vi "writeU16FIFO.vi"(8 "error in (no error)":errorcluster, 9 "Timeout":i32, 10 "Data":u16[](array[numeric]), 11 "ModbusSubnetETxDataFIFO in":refnum<class "ModbusSubnetETxDataFIFO.lvclass">) -> (0 "error out":errorcluster, 2 "ElementsRemaining":u32, 3 "ModbusSubnetETxDataFIFO out":refnum<class "ModbusSubnetETxDataFIFO.lvclass">)   [LabVIEW 2016, in "ModbusSubnetETxDataFIFO.lvclass"]
uses:
  ModbusSubnetETxDataFIFO.lvclass
  FPGA/FPGA.lvclass
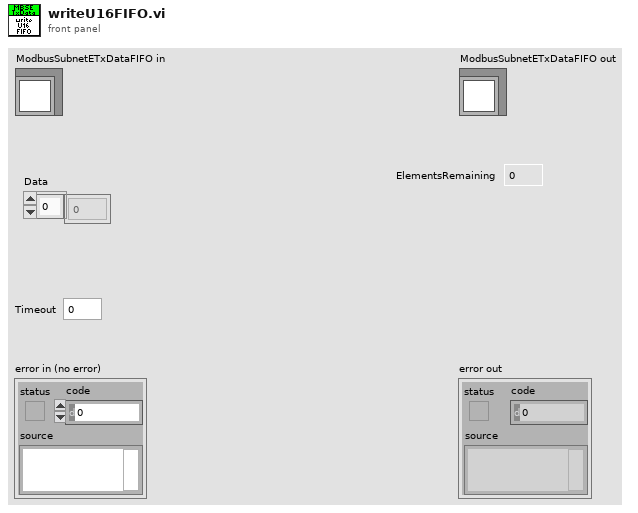
[diagram p1: front panel]
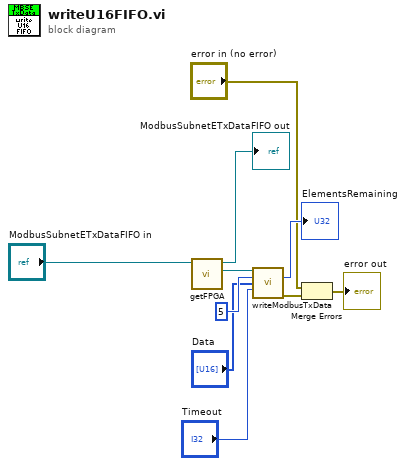
[diagram p0: block diagram]
diagram:
  n1 = call "getFPGA.vi"("ModbusSubnetETxDataFIFO in"="ModbusSubnetETxDataFIFO in") -> ("FPGA"=w9:refnum<class "FPGA.lvclass">, "ModbusSubnetETxDataFIFO out"=→"ModbusSubnetETxDataFIFO out":refnum<class "ModbusSubnetETxDataFIFO.lvclass">)  [unwired: 9 in]
  n2 = call "writeModbusTxData.vi"("FPGA in"=w9, 5:u16 5 ("Subnet"), 7:"Data", "Timeout (ms)"="Timeout") -> ("Empty Elements Remaining"=→"ElementsRemaining":u32, "error out"=w3:errorcluster)  [unwired: 9 in, 1 out]
  n3 = Merge Errors("error in (no error)", w3) -> (→"error out":errorcluster)
